vi "Unpack String.vi"(11 "Broadcast String Msg In":refnum<class "Broadcast String Msg.lvclass">) -> (2 "Value":string, 3 "Name":string)   [LabVIEW 2015, in "Broadcast String Msg.lvclass"]
uses:
  Broadcast String Msg.lvclass
  Broadcast String Msg.lvclass/Broadcast String Msg.ctl
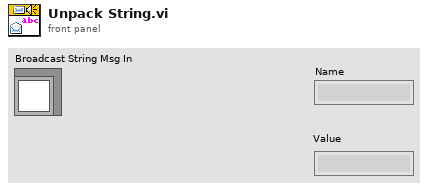
[diagram p1: front panel]
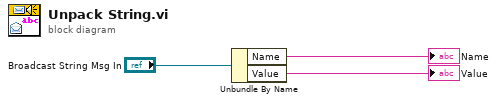
[diagram p0: block diagram]
diagram:
  n1 = Unbundle By Name("Broadcast String Msg In") -> ("Name"=→"Name":string, "Value"=→"Value":string)
